vi "Initialize.vi"(8 "error in (no error)":errorcluster, 10 "Logger information":T1={"Log File Path"="", "Verbosity"=enum."Default", "Append to log file?"=FALSE}, 11 "Logger in":refnum<class "Logger.lvclass">) -> (0 "error out":errorcluster, 3 "Logger out":refnum<class "Logger.lvclass">)   [LabVIEW 2014, in "Logger.lvclass"]
uses:
  Logger.lvclass
  LoggerCore.ctl
  Verbosity.ctl
  Logger.lvclass/Logger.ctl
  OperationErrorType.ctl
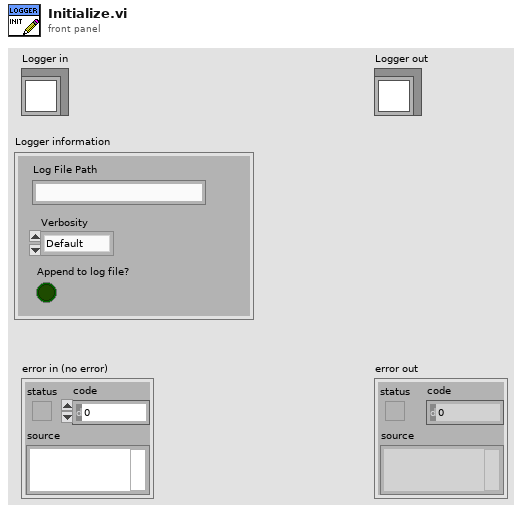
[diagram p1: front panel]
types:
  T1 = typedef "Logger.lvclass/LoggerCore.ctl" = cluster{"Log File Path":string, "Verbosity":T2, "Append to log file?":bool}
  T2 = typedef "Verbosity.ctl" = enum16{"Minimal", "Default", "Detailed", "Diagnostic"}
  T3 = typedef "OperationErrorType.ctl" = enum16{"RequiredArgumentMissing", "UnknownArguments", "LoggerSetMultipleTimes", "OperationBrokenError"}
  T4 = enum16{"open", "replace", "create", "open or create", "replace or create", "replace or create with confirmation"}
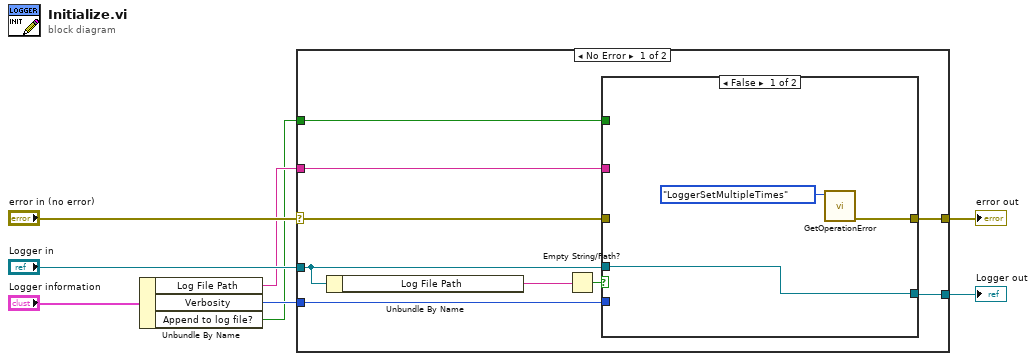
[diagram p0: block diagram]
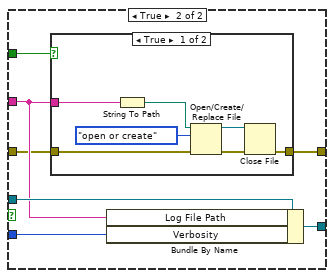
[diagram p2: hidden frame]
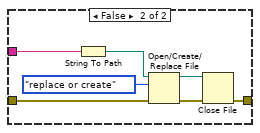
[diagram p3: hidden frame]
diagram:
  n1 = Unbundle By Name("Logger information") -> ("Log File Path"=w3:string, "Verbosity"=w2:T2, "Append to log file?"=w1:bool)
  n2 = case shown="No Error" "error in (no error)" {
    selector: "error in (no error)" -> [w15 w43]
    tunnel: [w14 w43] -> w8
    tunnel: [w16 w42] -> w6
    tunnel: "Logger in" -> [w10 w42]
    tunnel: w3 -> [w17 _]
    tunnel: w1 -> [w13 _]
    tunnel: w2 -> [w12 _]
    frame No Error {
      n3 = Unbundle By Name(w10) -> ("Log File Path"=w9:string)
      n4 = Empty String/Path?(string/path=w9) -> (empty?=w11:bool)
      n5 = case shown="False" w11 {
        tunnel: w17 -> [_ w25]
        tunnel: w10 -> [w20 w27]
        tunnel: [w20 w26] -> w16
        tunnel: w15 -> [_ w24]
        tunnel: [w18 w23] -> w14
        tunnel: w13 -> [_ w22]
        tunnel: w12 -> [_ w21]
        frame False {
          n6 = call "GetOperationError.vi"("Operation Error Type"=OperationErrorType."LoggerSetMultipleTimes") -> ("error out"=w18:errorcluster)  [unwired: 10 in]
        }
        frame True {
          n7 = case shown="True" w22 {
            tunnel: w25 -> [w34 w41]
            tunnel: [w30 w37] -> w23
            tunnel: w24 -> [w29 w36]
            frame True {
              n8 = String To Path(string=w34) -> (path=w28:path)
              n9 = Open/Create/Replace File(file path (use dialog)=w28, error in=w29, operation (0:open)=T4."open or create") -> (refnum out=w31:refnum<file>, error out=w32:errorcluster)  [unwired: 3 in, 1 out]
              n10 = Close File(refnum=w31, error in=w32) -> (error out=w30:errorcluster)  [unwired: 1 out]
            }
            frame False {
              n11 = String To Path(string=w41) -> (path=w35:path)
              n12 = Open/Create/Replace File(file path (use dialog)=w35, error in=w36, operation (0:open)=T4."replace or create") -> (refnum out=w38:refnum<file>, error out=w39:errorcluster)  [unwired: 3 in, 1 out]
              n13 = Close File(refnum=w38, error in=w39) -> (error out=w37:errorcluster)  [unwired: 1 out]
            }
          }
          n14 = Bundle By Name(cluster=w27, "Log File Path"=w25, "Verbosity"=w21) -> (w26:refnum<class "Logger.lvclass">)
        }
      }
    }
    frame Error {
    }
  }
  "error out" <- w8
  "Logger out" <- w6
